vi "RandomKastArrayBygger.vi"(0 "Andtal tærninger":dbl, 6 "Nedrre grænse":i32, 9 "Øvre grænse":i32, 10 "Array in":i32[](array[numeric]), 11 "Andtal kast":dbl) -> (3 "Array out":i32[](array[numeric]))   [LabVIEW 2022 SP3]
uses:
  <vilib>/numeric/Random Number (Range) U64.vi
  cf0dea72-97f7-4350-823b-c19a5e34ff0a.vi
  <vilib>/numeric/sub_Random U32.vi
panel:
  out "sum":u64
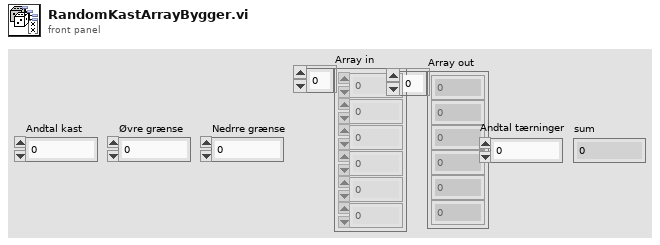
[diagram p1: front panel]
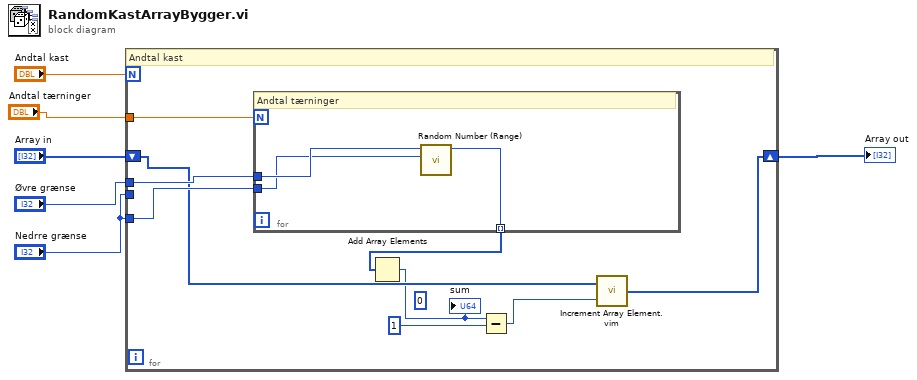
[diagram p0: block diagram]
diagram:
  n1 = for {
    N: "Andtal kast" -> [_]
    tunnel: "Øvre grænse" -> [w15]
    tunnel: "Nedrre grænse" -> [w14]
    tunnel: "Nedrre grænse" -> [_]
    shift-right: [w11] -> w2
    shift-left: "Array in" -> [w12]
    tunnel: "Andtal tærninger" -> [w7]
    (unwired) u64 0 ("sum")
    # "Andtal kast"
    n2 = for {
      N: w7 -> [_]
      tunnel: w15 -> [w18]
      tunnel: w14 -> [w17]
      tunnel: [w16] -> w10 mode=indexing
      # "Andtal tærninger"
      n3 = call-poly <vilib>:"Random Number (Range).vi"("lower bound (0)"=w17, "upper bound (100)"=w18) -> ("number"=w16:u64)  [unwired: 9 in]
    }
    n4 = Add Array Elements(numeric array=w10) -> (sum=w8:u64)
    "sum" <- w8
    n5 = Subtract(x=w8, y=i64 1) -> (x-y=w13:u64)
    n6 = call "Increment Array Element.vim"("index"=w13, "array in"=w12) -> ("array out"=w11:i32[])
  }
  "Array out" <- w2
